vi "Replace_Array_Subset_2D_SubArray.vi"(9 "SubArray RAS2D":i8[](array[numeric]), 10 "Indexs RAS2D":T1={"Rows"=-1, "Columns"=-1} {"Columns" min=-1; "Rows" min=-1}, 11 "RAS2D":i8[][](array[numeric])) -> (3 "New Array RAS2D":i8[][](array[numeric]))   [LabVIEW 2018]
uses:
  Controls/Rows_Columns.ctl
panel:
  out "Size":i32
  out "IC":i32
  out "IR":i32
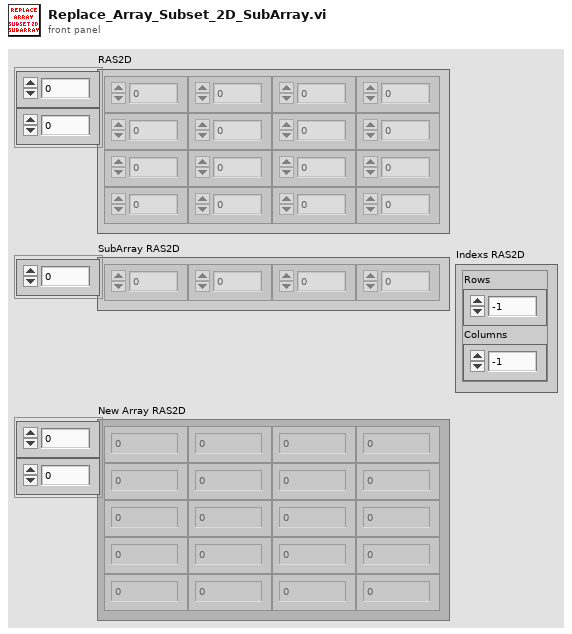
[diagram p1: front panel]
types:
  T1 = typedef "Rows_Columns.ctl" = cluster{"Rows":i32, "Columns":i32}
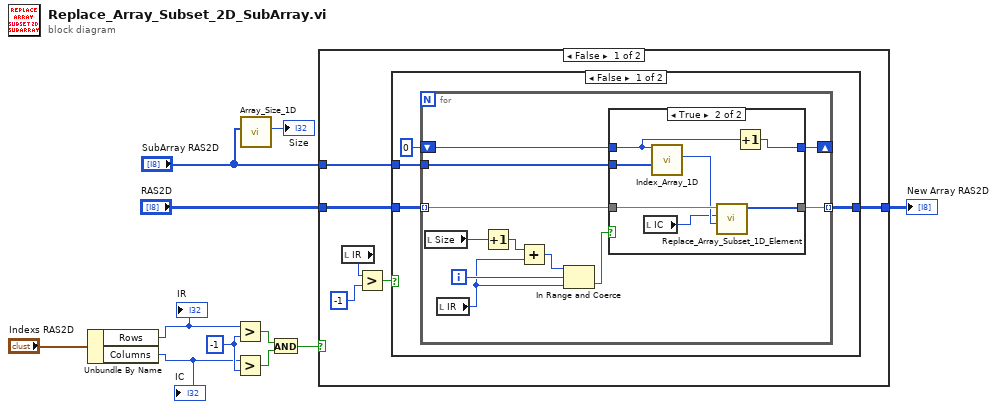
[diagram p0: block diagram]
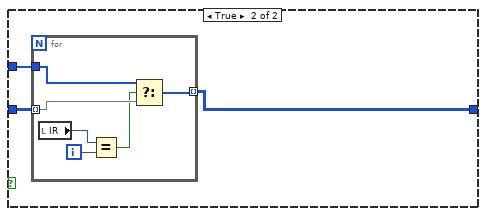
[diagram p3: hidden frame]
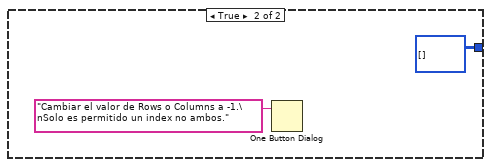
[diagram p4: hidden frame]
diagram:
  w7 = -1 ("y")
  n1 = Unbundle By Name("Indexs RAS2D") -> ("Rows"=w5:i32, "Columns"=w4:i32)
  "IR" <- w5
  "IC" <- w4
  n2 = Greater?(x=w5, y=w7) -> (0:w9:bool)
  n3 = Greater?(x=w4, y=w7) -> (0:w8:bool)
  n4 = call "Array_Size_1D.vi"("Array"="SubArray RAS2D") -> ("Size"=→"Size":i32)  [unwired: 10 in]
  n5 = And(x=w9, y=w8) -> (x .and. y?=w10:bool)
  n6 = case shown="False" w10 {
    tunnel: "RAS2D" -> [w17 _]
    tunnel: "SubArray RAS2D" -> [w16 _]
    tunnel: [w12 i8[][] [] ("RAS2D")] -> w1
    frame False {
      n7 = local read "IR"() -> (w14:i32)
      n8 = Greater?(x=w14, y=-1) -> (0:w13:bool)
      n9 = case shown="False" w13 {
        tunnel: w17 -> [w20 w44]
        tunnel: w16 -> [w21 w43]
        tunnel: [w18 w42] -> w12
        frame False {
          n10 = for {
            tunnel: w21 -> [w31]
            tunnel: w20 -> [w32] mode=indexing
            shift-right: [w30] -> _
            shift-left: 0 ("y") -> [w29]
            tunnel: [w28] -> w18 mode=indexing
            i -> [w26]
            n11 = local read "Size"() -> (w25:i32)
            n12 = local read "IR"() -> (w24:i32)
            n13 = Increment(x=w25) -> (x+1=w22:i32)
            n14 = Add(x=w22, y=w24) -> (x+y=w23:i32)
            n15 = In Range and Coerce(upper limit=w23, x=w26, lower limit=w24) -> (In Range?=w27:bool)  [unwired: 1 out]
            n16 = case shown="True" w27 {
              tunnel: w32 -> [w34 w41]
              tunnel: w31 -> [_ w40]
              tunnel: [w33 w37] -> w30
              tunnel: w29 -> [w33 w36]
              tunnel: [w34 w35] -> w28
              frame False {
              }
              frame True {
                n17 = local read "IC"() -> (w38:i32)
                n18 = call "Index_Array_1D.vi"("Index Array 1D"=w40, "Index"=w36) -> ("Value"=w39:i8)  [unwired: 9 in]
                n19 = call "Replace_Array_Subset_1D_Element.vi"("Element RAS"=w39, "Index RAS1D"=w38, "RAS1D"=w41) -> ("New Array RAS1D"=w35:i8[])  [unwired: 8 in]
                n20 = Increment(x=w36) -> (x+1=w37:i32)
              }
            }
          }
        }
        frame True {
          n21 = for {
            tunnel: w44 -> [w50] mode=indexing
            tunnel: [w49] -> w42 mode=indexing
            tunnel: w43 -> [w46]
            i -> [w47]
            n22 = local read "IR"() -> (w48:i32)
            n23 = Equal?(x=w48, y=w47) -> (x = y?=w45:bool)
            n24 = Select(t=w46, s=w45, f=w50) -> (s? t:f=w49:i8[])
          }
        }
      }
    }
    frame True {
      n25 = One Button Dialog(message="Cambiar el valor de Rows o Columns a -1.\nSolo es permitido un index no ambos.") -> ()  [unwired: 1 in, 1 out]
    }
  }
  "New Array RAS2D" <- w1
